vi "p2.vi"() -> ()   [LabVIEW 2023, in "d6.lvlib"]
uses:
  d6.lvlib
  <vilib>/Utility/error.llb/Trim Whitespace One-Sided.vi
  <vilib>/Analysis/polynomials.llb/Polynomial Roots (DBL).vi
  <vilib>/regexp/Match Regular Expression.xnode
  AOC/AOC.lvlib
  <vilib>/Analysis/NI_AALPro.lvlib
panel:
  in  "Input":string="Time:        35     69     68     87\nDistance:   213   1168   1086   1248"
  in  "Example":string="Time:      7  15   30\nDistance:  9  40  200"
  in  "Example":bool=TRUE
  out "Answer":i64=1909
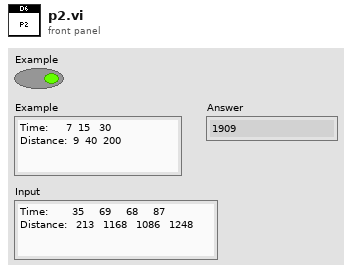
[diagram p1: front panel]
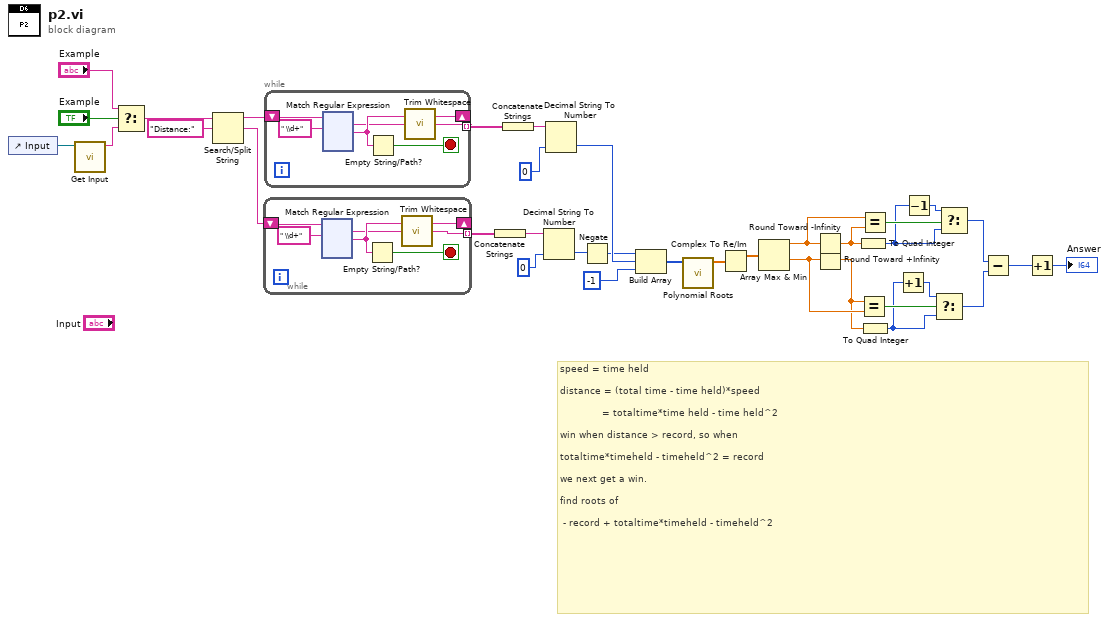
[diagram p0: block diagram]
diagram:
  # "speed = time held\n\ndistance = (total time - time held)*speed\n\n              = totaltime*time held - time held^2\n\nwin when distance > record, so when \n\ntotaltime*timeheld - timeheld^2 = record\n\nwe next get a win.\n\nfind roots of\n\n - record + totaltime*timeheld - timeheld^2"
  n1 = control-ref of="Input"() -> (w1:refnum<vi>)
  n2 = call "Get Input.vi"("Input ref"=w1) -> ("Input"=w35:string)  [unwired: 10 in]
  n3 = Select(t="Example", s="Example", f=w35) -> (s? t:f=w32:string)
  n4 = Search/Split String(string=w32, search string/char (-)="Distance:") -> (substring before match=w30:string, match + rest of string=w29:string)  [unwired: 1 in, 1 out]
  n5 = while {
    tunnel: [w36] -> w28 mode=indexing
    shift-right: [w38] -> _
    shift-left: w29 -> [w41]
    stop <- w39 stop-if-true
    n6 = xnode "Match Regular Expression"("input string"=w41, "regular expression"=" \\d+") -> ("whole match"=w37:string, "after match"=w38:string)  [unwired: 4 in, 3 out]
    n7 = Empty String/Path?(string/path=w38) -> (empty?=w39:bool)
    n8 = call <vilib>:"Trim Whitespace.vi"("string"=w37) -> ("trimmed string"=w36:string)  [unwired: 1 in]
  }
  n9 = while {
    tunnel: [w159] -> w4 mode=indexing
    shift-right: [w161] -> _
    shift-left: w30 -> [w164]
    stop <- w162 stop-if-true
    n10 = xnode "Match Regular Expression"("input string"=w164, "regular expression"=" \\d+") -> ("whole match"=w160:string, "after match"=w161:string)  [unwired: 4 in, 3 out]
    n11 = Empty String/Path?(string/path=w161) -> (empty?=w162:bool)
    n12 = call <vilib>:"Trim Whitespace.vi"("string"=w160) -> ("trimmed string"=w159:string)  [unwired: 1 in]
  }
  n13 = Concatenate Strings(w28) -> (w3:string)
  n14 = Concatenate Strings(w4) -> (w2:string)
  n15 = Decimal String To Number(string=w3, default (0L)=i64 0 ("Answer")) -> (number=w24:i64)  [unwired: 1 in, 1 out]
  n16 = Decimal String To Number(string=w2, default (0L)=i64 0 ("Answer")) -> (number=w25:i64)  [unwired: 1 in, 1 out]
  n17 = Negate(x=w24) -> (-x=w22:i64)
  n18 = Build Array(w22, w25, i64 -1 ("element")) -> (w20:i64[])
  n19 = call-poly <vilib>:"Polynomial Roots.vi"("P(x)"=w20) -> ("Roots"=w19:cdb[])  [unwired: 9 in, 1 out]
  n20 = Complex To Re/Im(x + iy=w19) -> (x=w18:dbl[])  [unwired: 1 out]
  n21 = Array Max & Min(array=w18) -> (max value=w16:dbl, min value=w17:dbl)  [unwired: 2 out]
  n22 = Round Toward -Infinity(1:w16) -> (0:w11:dbl)
  n23 = Round Toward +Infinity(x=w17) -> (ceil(x): smallest int >= x=w9:dbl)
  n24 = To Quad Integer(1:w11) -> (0:w10:i64)
  n25 = Equal?(x=w9, y=w17) -> (x = y?=w15:bool)
  n26 = Equal?(x=w16, y=w11) -> (x = y?=w13:bool)
  n27 = To Quad Integer(1:w9) -> (0:w8:i64)
  n28 = Increment(x=w8) -> (x+1=w14:i64)
  n29 = Decrement(x=w10) -> (x-1=w12:i64)
  n30 = Select(t=w14, s=w15, f=w8) -> (s? t:f=w6:i64)
  n31 = Select(t=w12, s=w13, f=w10) -> (s? t:f=w7:i64)
  n32 = Subtract(x=w7, y=w6) -> (x-y=w5:i64)
  n33 = Increment(x=w5) -> (x+1=→"Answer":i64)
